vi "Example.vi"(2 "Debug Mode":bool, 3 "Elapsed Time (s)":dbl, 4 "State":enum16{"Edit", "Start", "Run", "End", "Idle"}(ring), 5 "Argument List In":string[](array[string])) -> (0 "Status Out":string, 1 "Argument List Out":string[](array[string]))   [LabVIEW 2011]
panel:
  in  "Parameter 3":dbl
  in  "Cancel":bool
  in  "Parameter 1":bool
  in  "Parameter 2":string
  in  "OK":bool
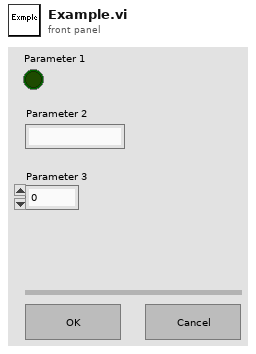
[diagram p1: front panel]
types:
  T1 = enum16{"Discrete", "Continuous", "Instantaneous"}
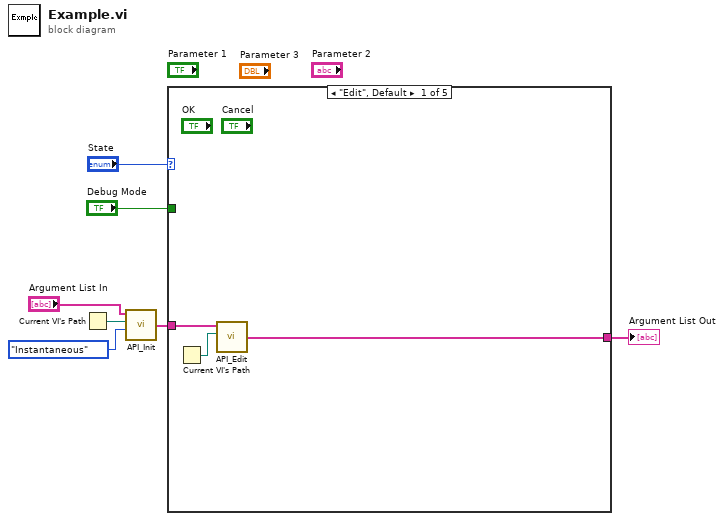
[diagram p0: block diagram]
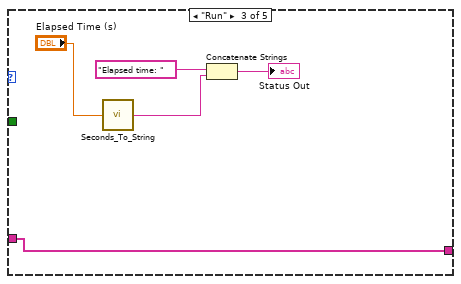
[diagram p3: hidden frame]
diagram:
  n1 = Current VI's Path() -> (path=w3:path)
  n2 = call "API_Init.vi"("API Mode"=T1."Instantaneous", "VI Path"=w3, "Argument List In"="Argument List In") -> ("Argument List Out"=w4:string[])  [unwired: 1 in]
  n3 = case shown="\"Edit\", Default" "State" {
    tunnel: [w8 w11 w12 w17 w18] -> w6
    tunnel: w4 -> [w10 w11 w12 w17 w18]
    tunnel: "Debug Mode" -> [_ _ _ _ _]
    frame "Edit", Default {
      n4 = Current VI's Path() -> (path=w9:path)
      n5 = call "API_Edit.vi"("VI Path"=w9, "Argument List In"=w10) -> ("Argument List Out"=w8:string[])  [unwired: 2 in]
    }
    frame "Start" {
    }
    frame "Run" {
      n6 = call "Seconds_To_String.vi"("Seconds"="Elapsed Time (s)") -> ("Output String"=w14:string)
      n7 = Concatenate Strings("Elapsed time: " ("string"), w14) -> (→"Status Out":string)
    }
    frame "End" {
    }
    frame "Idle" {
    }
  }
  "Argument List Out" <- w6
